vi "Load DAC Configuration.vi"(8 "error in":errorcluster, 10 "Config File refnum in":T1, 11 "DAC Keller BNC in":refnum<class "DAC Keller BNC.lvclass">) -> (0 "error out":errorcluster, 2 "Config File refnum out":T1, 3 "DAC Keller BNC out":refnum<class "DAC Keller BNC.lvclass">)   [LabVIEW 2019, in "DAC.lvlib" / "DAC Keller BNC.lvclass"]
uses:
  DAC Keller BNC.lvclass
  DAC.lvclass
  <vilib>/Utility/config.llb/NI_LVConfig.lvlib
  <vilib>/Utility/config.llb/Read Key (I32).vi
  <vilib>/Utility/config.llb/Read Key (String).vi
  C:/Users/krio/Documents/LV_Projects/test-stand/App/DAC/DAC.lvclass
  <vilib>/Utility/config.llb/Config Data RefNum.ctl
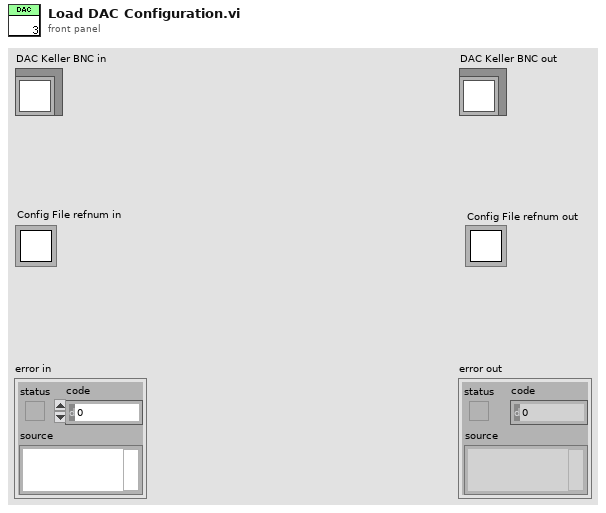
[diagram p1: front panel]
types:
  T1 = typedef "NI_LVConfig.lvlib/Config Data RefNum.ctl" = refnum<k1>
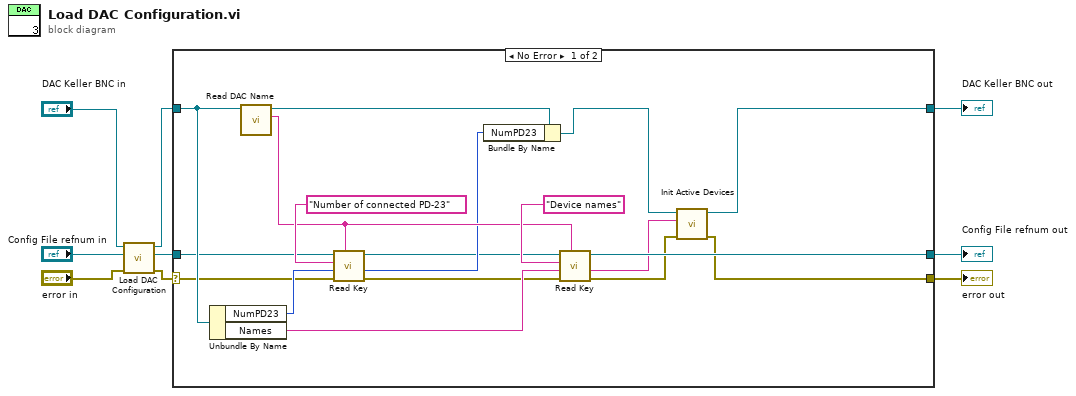
[diagram p0: block diagram]
diagram:
  n1 = call-parent "Load DAC Configuration.vi"("error in"="error in", "Config File refnum in"="Config File refnum in", "DAC in"="DAC Keller BNC in") -> ("error out"=w4:errorcluster, "Config File refnum out"=w5:T1, "DAC out"=w6:refnum<class "DAC Keller BNC.lvclass">)  [unwired: 6 in]
  n2 = case shown="No Error" w4 {
    selector: w4 -> [w12 w30]
    tunnel: [w19 w30] -> w1
    tunnel: [w22 w29] -> w3
    tunnel: w6 -> [w25 w29]
    tunnel: w5 -> [w13 w28]
    tunnel: [w27 w28] -> w2
    frame No Error {
      n3 = Unbundle By Name(w25) -> ("NumPD23"=w16:i32, "Names"=w24:string)
      n4 = call "Read DAC Name.vi"("DAC in"=w25) -> ("DAC Name"=w17:string, "DAC out"=w23:refnum<class "DAC Keller BNC.lvclass">)  [unwired: 8 in, 1 out]
      n5 = call-poly <vilib>:"Read Key.vi"("section"=w17, "error in (no error)"=w12, "default value"=w16, "key"="Number of connected PD-23", "refnum"=w13) -> ("error out"=w10:errorcluster, "value"=w14:i32, "refnum out"=w11:T1)  [unwired: 3 in, 1 out]
      n6 = Bundle By Name(cluster=w23, "NumPD23"=w14) -> (w15:refnum<class "DAC Keller BNC.lvclass">)
      n7 = call-poly <vilib>:"Read Key.vi"("section"=w17, "error in (no error)"=w10, "default value"=w24, "key"="Device names", "refnum"=w11) -> ("error out"=w20:errorcluster, "value"=w21:string, "refnum out"=w27:T1)  [unwired: 3 in, 1 out]
      n8 = call "Init Active Devices.vi"("error in"=w20, "Device Names"=w21, "DAC Keller BNC in"=w15) -> ("error out"=w19:errorcluster, "DAC Keller BNC out"=w22:refnum<class "DAC Keller BNC.lvclass">)  [unwired: 7 in]
    }
    frame Error {
    }
  }
  "error out" <- w1
  "DAC Keller BNC out" <- w3
  "Config File refnum out" <- w2
